vi "Opposing Direction.vi"(10 "Direction":T1) -> (2 "Opposing Direction":T1)   [LabVIEW 2020, in "SquareBattle.lvlib"]
uses:
  SquareBattle.lvlib
  Direction.ctl
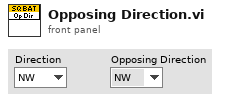
[diagram p1: front panel]
types:
  T1 = typedef "SquareBattle.lvlib/Direction.ctl" = enum16{"NW", "N", "NE", "E", "SE", "S", "SW", "W"}
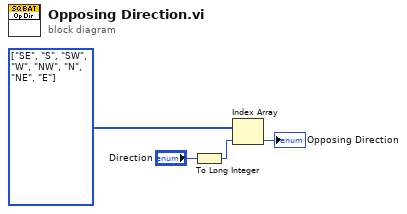
[diagram p0: block diagram]
diagram:
  w4 = T1[] [enum."SE", enum."S", enum."SW", enum."W", enum."NW", enum."N", enum."NE", enum."E"] items=["NW", "N", "NE", "E", "SE", "S", "SW", "W"]
  n1 = To Long Integer(number="Direction") -> (32bit integer=w1:i32)
  n2 = Index Array(array=w4, index=w1) -> (element=→"Opposing Direction":T1)
